vi "Keyboard.vi"() -> ()   [LabVIEW 2012]
doc: "if you need more information write at urieluribe@hotmail.com"
uses:
  <vilib>/Utility/inputDevices.llb/keyboardAcquire.vi
panel:
  out "key":T1(ring)
  out "String":string
  in  "stop":bool
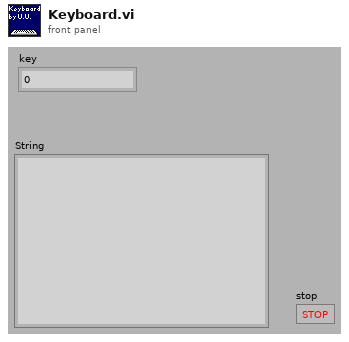
[diagram p1: front panel]
types:
  T1 = enum16{"0", "1", "2", "3", "4", "5", "6", "7", "8", "9", "A", "B", "C", "D", "E", "F", "G", "H", "I", "J", "K", "L", "M", "N", "O", "P", "Q", "R", "S", "T", "U", "V", "W", "X", "Y", "Z", "F1", "F2", "F3", "F4", "F5", "F6", "F7", "F8", "F9", "F10", "F11", "F12", "F13", "F14", "F15", "ADD", "BACK", "BACKSLASH", "CAPITAL", "COMMA", "DECIMAL", "DELETE", "DIVIDE", "DOWN", "END", "EQUALS", "ESCAPE", "GRAVE (`)", "HOME", "INSERT", "LBRACKET", "LCONTROL", "LEFT", "L ALT", "LSHIFT", "LWIN", "MINUS", "MULTIPLY", "NEXT", "NUMLOCK", "NUMPAD_0", "NUMPAD_1", "NUMPAD_2", "NUMPAD_3", "NUMPAD_4", "NUMPAD_5", "NUMPAD_6", "NUMPAD_7", "NUMPAD_8", "NUMPAD_9", "PAUSE", "PERIOD", "PRIOR (PG UP)", "RBRACKET", "RCONTROL", "RETURN", "RIGHT", "R ALT", "RSHIFT", "RWIN", "SCROLL", "SEMICOLON", "SLASH", "SPACE", "SUBTRACT", "TAB", "UP", "ENTER (num pad)", "' (quote)"}
  T2 = enum16{"0", "1", "2", "3", "4", "5", "6", "7", "8", "9", "A", "B", "C", "D", "E", "F", "G", "H", "I", "J", "K", "L", "M", "N", "O", "P", "Q", "R", "S", "T", "U", "V", "W", "X", "Y", "Z", "F1", "F2", "F3", "F4", "F5", "F6", "F7", "F8", "F9", "F10", "F11", "F12", "F13", "F14", "F15", "ADD", "BACK", "BACKSLASH", "CAPITAL", "COMMA", "DECIMAL", "DELETE", "DIVIDE", "DOWN", "END", "EQUALS", "ESCAPE", "GRAVE (`)", "HOME", "INSERT", "LBRACKET", "LCONTROL", "LEFT", "L ALT", "LSHIFT", "LWIN", "MINUS", "MULTIPLY", "NEXT", "NUMLOCK", "NUMPAD_0", "NUMPAD_1", "NUMPAD_2", "NUMPAD_3", "NUMPAD_4", "NUMPAD_5", "NUMPAD_6", "NUMPAD_7", "NUMPAD_8", "NUMPAD_9", "PAUSE", "PERIOD", "PRIOR (PG UP)", "RBRACKET", "RCONTROL", "RETURN", "RIGHT", "R ALT", "RSHIFT", "RWIN", "SCROLL", "SEMICOLON", "SLASH", "SPACE", "SUBTRACT", "TAB", "UP", "ENTER (num pad)", "' (quote)"}[]
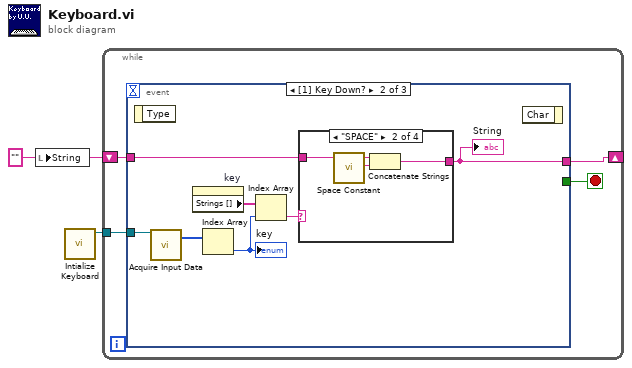
[diagram p0: block diagram]
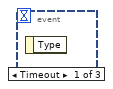
[diagram p2: hidden frame]
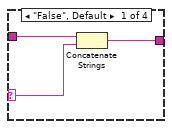
[diagram p3: hidden frame]
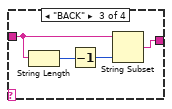
[diagram p4: hidden frame]
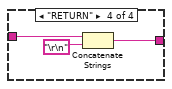
[diagram p5: hidden frame]
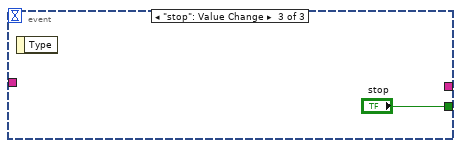
[diagram p6: hidden frame]
diagram:
  w1 = ""
  n1 = local write "String"(w1) -> ()
  n2 = call <vilib>:"Intialize Keyboard.vi"() -> ("device ID"=w2:refnum<k1>)  [unwired: 10 in, 1 out]
  n3 = while {
    tunnel: w2 -> [w5]
    shift-right: [w4] -> _
    shift-left: w1 -> [w3]
    stop <- w6 stop-if-true
    n4 = event shown="[1] Key Down?" {
      selector: _ -> [_ _ _]
      dyn-events: _ -> [_ _ _]
      timeout: _ -> [_ _ _]
      tunnel: [_ _ "stop"] -> w6
      tunnel: w5 -> [_ w13 _]
      tunnel: [_ w7 _] -> w4
      tunnel: w3 -> [_ w8 _]
      event Timeout {
        n5 = event-data() -> ()  [unwired: 1 in, 1 out]
      }
      event Key Down? {
        n6 = event-data() -> ()  [unwired: 1 in, 1 out]
        n7 = call-poly <vilib>:"Acquire Input Data.vi"("device ID"=w13) -> ("keys pressed"=w12:T2)  [unwired: 16 in, 2 out]
        n8 = property on="key" class="Enum (strict)"() -> ("Strings []"=w10:string[])  [unwired: 2 in, 2 out]
        n9 = Index Array(array=w12) -> (element=w11:T1)  [unwired: 1 in]
        "key" <- w11
        n10 = Index Array(array=w10, index=w11) -> (element=w9:string)
        n11 = case shown="\"SPACE\"" w9 {
          selector: w9 -> [w14 _ _ _]
          tunnel: w8 -> [w16 w19 w23 w26]
          tunnel: [w15 w17 w21 w24] -> w7
          frame "False", Default {
            n12 = Concatenate Strings(w16, w14) -> (w15:string)
          }
          frame "SPACE" {
            n13 = call <vilib>:"Space Constant.vi"() -> ("String"=w18:string)
            n14 = Concatenate Strings(w19, w18) -> (w17:string)
          }
          frame "BACK" {
            n15 = String Length(string=w23) -> (length=w22:i32)
            n16 = Decrement(x=w22) -> (x-1=w20:i32)
            n17 = String Subset(string=w23, length (rest)=w20) -> (substring=w21:string)  [unwired: 1 in]
          }
          frame "RETURN" {
            n18 = Concatenate Strings(w26, "\r\n") -> (w24:string)
          }
        }
        "String" <- w7
        n19 = event-data() -> ()  [unwired: 2 in, 1 out]
      }
      event "stop": Value Change {
        n20 = event-data() -> ()  [unwired: 1 in, 1 out]
      }
    }
  }
